vi "Init.vi"(8 "error in (no error)":errorcluster, 10 "Channel":i16, 11 "TrialBasedExperiment in":refnum<class "DotMappingExperiment.lvclass">) -> (0 "error out":errorcluster, 3 "TrialBasedExperiment out":refnum<class "DotMappingExperiment.lvclass">)   [LabVIEW 2014, in "DotMappingExperiment.lvclass"]
uses:
  DotMappingExperiment.lvclass
  Trial Based Experiment Statechart/PassiveExperiment/PassiveExperiment.lvclass
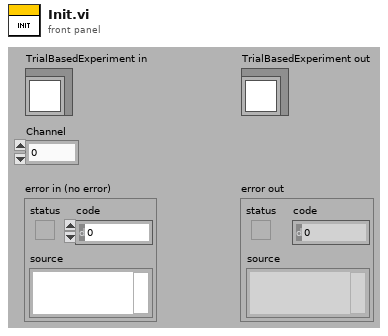
[diagram p1: front panel]
types:
  T1 = cluster{"Intertrial":dbl, "AcquireFixation":dbl, "HoldFixation":dbl, "DelayPeriod":dbl, "ResponsePeriod":dbl}
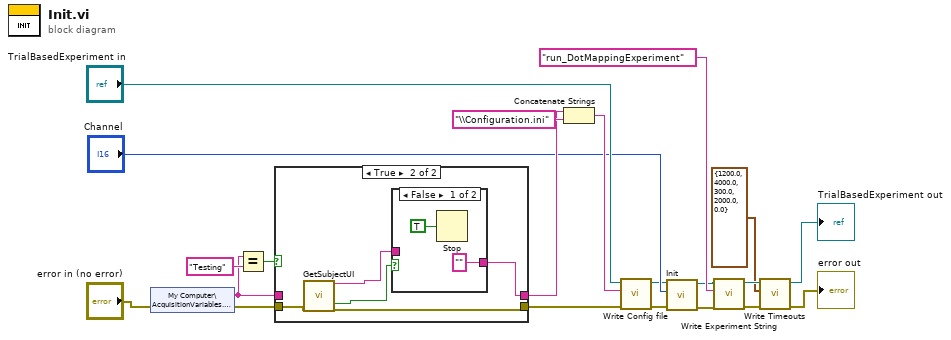
[diagram p0: block diagram]
diagram:
  n1 = shared-variable "My Computer\\AcquisitionVariables.lvlib\\Subject"(error in="error in (no error)") -> (w15:string, error out=w14:errorcluster)
  n2 = Equal?(x=w15, y="Testing") -> (x = y?=w17:bool)
  n3 = case shown="True" w17 {
    tunnel: [w23 w28] -> w10
    tunnel: w15 -> [w23 _]
    tunnel: w14 -> [w22 w24]
    tunnel: [w22 w25] -> w13
    frame False {
    }
    frame True {
      n4 = call "GetSubjectUI.vi"("error in (no error)"=w24) -> ("subjectSelected"=w27:string, "OK"=w26:bool, "error out"=w25:errorcluster)  [unwired: 16 in]
      n5 = case shown="False" w26 {
        tunnel: w27 -> [_ w31]
        tunnel: ["" ("subjectSelected") w31] -> w28
        frame False {
          n6 = Stop(stop? (T)=TRUE) -> ()
        }
        frame True {
        }
      }
    }
  }
  n7 = Concatenate Strings(w10, "\\Configuration.ini") -> (w19:string)
  n8 = call-dynamic "Write Config file.vi"("error in (no error)"=w13, "Config file"=w19, "TrialBasedExperiment in"="TrialBasedExperiment in") -> ("error out"=w5:errorcluster, "TrialBasedExperiment out"=w6:refnum<class "DotMappingExperiment.lvclass">)  [unwired: 7 in]
  n9 = call-parent "Init.vi"("error in (no error)"=w5, "Channel"="Channel", "TrialBasedExperiment in"=w6) -> ("error out"=w3:errorcluster, "TrialBasedExperiment out"=w4:refnum<class "DotMappingExperiment.lvclass">)  [unwired: 7 in]
  n10 = call-dynamic "Write Experiment String.vi"("error in (no error)"=w3, "Experiment String"="run_DotMappingExperiment" ("string"), "TrialBasedExperiment in"=w4) -> ("error out"=w20:errorcluster, "TrialBasedExperiment out"=w21:refnum<class "DotMappingExperiment.lvclass">)  [unwired: 7 in]
  n11 = call-dynamic "Write Timeouts.vi"("error in (no error)"=w20, "Timeouts"=T1 {"Intertrial"=1200.0, "AcquireFixation"=4000.0, "HoldFixation"=300.0, "DelayPeriod"=2000.0, "ResponsePeriod"=0.0}, "TrialBasedExperiment in"=w21) -> ("error out"=→"error out":errorcluster, "TrialBasedExperiment out"=→"TrialBasedExperiment out":refnum<class "DotMappingExperiment.lvclass">)  [unwired: 7 in]
